vi "加速度_绝对值-均值.vi"(11 "信号X":dbl[](array[numeric])) -> (3 "均值":dbl)   [LabVIEW 2014]
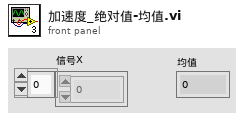
[diagram p1: front panel]
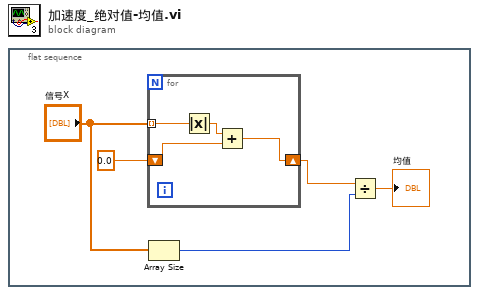
[diagram p0: block diagram]
diagram:
  n1 = flat-sequence {
    frame #0 {
      n2 = for {
        tunnel: "信号X" -> [w9] mode=indexing
        shift-right: [w6] -> w3
        shift-left: 0.0 -> [w7]
        n3 = Absolute Value(x=w9) -> (abs(x)=w8:dbl)
        n4 = Add(x=w8, y=w7) -> (x+y=w6:dbl)
      }
      n5 = Array Size(array="信号X") -> (size(s)=w2:i32)
      n6 = Divide(x=w3, y=w2) -> (x/y=→"均值":dbl)
    }
  }
